vi "DHE_DRV_get_actual_inttime.vi"(11 "error in (no error)":errorcluster) -> (8 "actual inttime":i32, 10 "supported":bool, 15 "error out":errorcluster)   [LabVIEW 2016]
doc: "This VI closes the I/O interface with the instrument."
uses:
  c/lib/libarcDHE.so
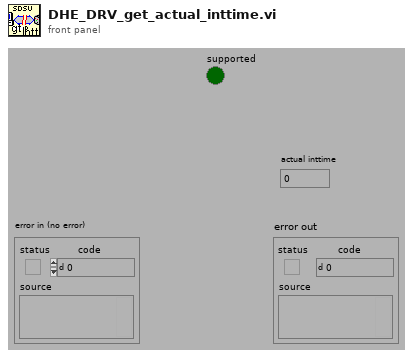
[diagram p1: front panel]
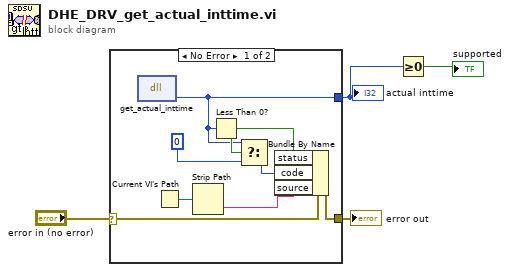
[diagram p0: block diagram]
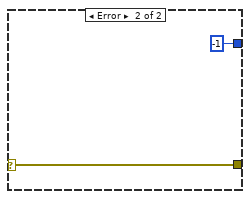
[diagram p2: hidden frame]
diagram:
  n1 = case shown="No Error" "error in (no error)" {
    selector: "error in (no error)" -> [w9 w13]
    tunnel: [w6 -1] -> w2
    tunnel: [w10 w13] -> w4
    frame No Error {
      n2 = dll-call lib="home/simager/panview/PAN/Modules/SDSU/private/c/lib/libarcDHE.so" fn="get_actual_inttime" label="read_actual_inttime"() -> ("return type"=w6:i32)  [unwired: 3 in, 2 out]
      n3 = Current VI's Path() -> (path=w12:path)
      n4 = Strip Path(path=w12) -> (name=w11:string)  [unwired: 1 out]
      n5 = Less Than 0?(x=w6) -> (x < 0?=w8:bool)
      n6 = Select(t=w6, s=w8, f=0) -> (s? t:f=w7:i32)
      n7 = Bundle By Name(cluster=w9, "status"=w8, "code"=w7, "source"=w11) -> (w10:errorcluster)
    }
    frame Error {
    }
  }
  "error out" <- w4
  "actual inttime" <- w2
  n8 = Greater Or Equal To 0?(x=w2) -> (x >= 0?=→"supported":bool)
